vi "Demo.vi"() -> ()   [LabVIEW 2017]
uses:
  Components/ViPER.lvlibp/ViPER.lvclass
panel:
  in  "stop":bool
  in  "Config XML":string="<?xml version=\"1.0\" encoding=\"UTF-8\" standalone=\"no\" ?>\n<Object>\n\n  <Name>Barcode</Name>\n\n  <Class>QR_Reader_Sim</Class>\n</Object>\n"
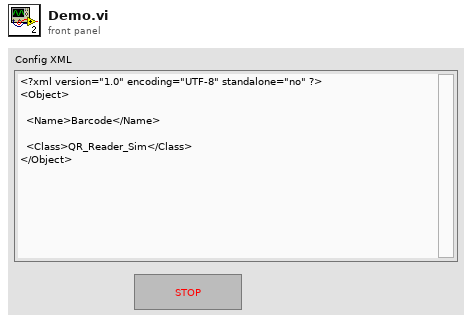
[diagram p1: front panel]
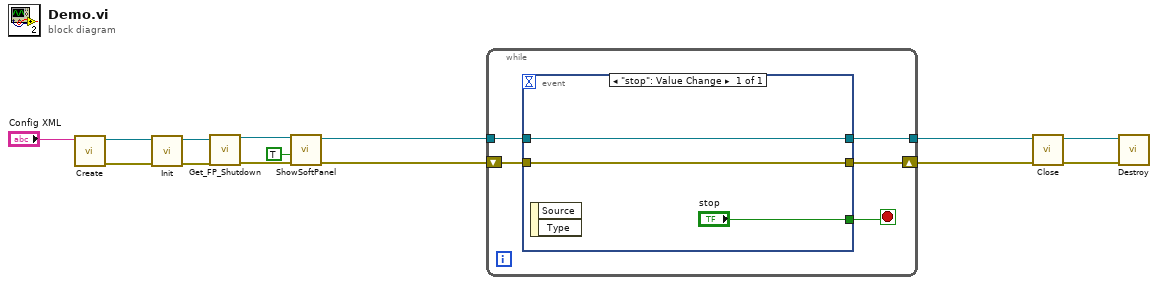
[diagram p0: block diagram]
diagram:
  n1 = call "Create.vi"("Config XML"="Config XML") -> ("error out"=w14:errorcluster, "reference out"=w13:refnum<class "ViPER.lvclass">)  [unwired: 9 in]
  n2 = call-dynamic "Init.vi"("error in (no error)"=w14, "reference in"=w13) -> ("error out"=w11:errorcluster, "reference out"=w10:refnum<class "ViPER.lvclass">)  [unwired: 8 in]
  n3 = call "Get_FP_Shutdown.vi"("ViKing_Base in"=w10, "error in (no error)"=w11) -> ("ViKing_Base out"=w8:refnum<class "ViPER.lvclass">, "error out"=w9:errorcluster)  [unwired: 9 in, 3 out]
  n4 = call-dynamic "ShowSoftPanel.vi"("error in (no error)"=w9, "Floating"=TRUE, "Driver in"=w8) -> ("error out"=w1:errorcluster, "Driver out"=w5:refnum<class "ViPER.lvclass">)  [unwired: 6 in, 1 out]
  n5 = while {
    tunnel: w5 -> [w18]
    shift-right: [w16] -> w3
    shift-left: w1 -> [w19]
    tunnel: [w15] -> w4
    stop <- w17 stop-if-true
    n6 = event shown="[0] \"stop\": Value Change" {
      selector: _ -> [_]
      dyn-events: _ -> [_]
      timeout: _ -> [_]
      tunnel: w19 -> [w21]
      tunnel: w18 -> [w20]
      tunnel: ["stop"] -> w17
      tunnel: [w21] -> w16
      tunnel: [w20] -> w15
      event "stop": Value Change {
        n7 = event-data() -> ()  [unwired: 1 in, 2 out]
      }
    }
  }
  n8 = call-dynamic "Close.vi"("error in (no error)"=w3, "reference in"=w4) -> ("error out"=w7:errorcluster, "reference out"=w6:refnum<class "ViPER.lvclass">)  [unwired: 8 in]
  n9 = call "Destroy.vi"("error in (no error)"=w7, "reference in"=w6) -> ()  [unwired: 9 in, 1 out]
